vi "Point To Row Column.vi"(8 "error in (no error)":errorcluster, 10 "Point":T2, 11 "DigitalTable in":refnum<class "DigitalTable.lvclass">) -> (0 "error out":errorcluster, 1 "Cell Position":T1, 2 "In Bounds?":bool, 3 "DigitalTable out":refnum<class "DigitalTable.lvclass">)   [LabVIEW 2023, in "DigitalTable.lvclass"]
doc: "Converts a pixel coordinate to a row-column pair in the coordinates of the control. This method also returns whether the point is inside the bounds of the content rectangle.\n\n <b>Note</b> The Point to Row Column method does not return an error for points that lie within a control but outside of the actual cell area for that control, such as the scroll bar. Use the InBounds parameter to verify that a point lies within the cell area of a control.\n\nQControl Class wrapper around the <b>DigitalTable : Point to Row Column Method</b>.\n<b> </b> <b> </b>\n©2016 Q Software Innovations, LLC (QSI)\nwritten by Quentin Alldredge\nproduced in LabVIEW 2015\n\nsupport@qsoftwareinnovations.com\nwww.qsoftwareinnovations.com\n\nAll rights reserved.\n\nRedistribution and use in source and binary forms, with or without modification, are permitted provided that the following conditions are met:\n\n * Redistributions of source code must retain the above copyright notice, this list of conditions and the following disclaimer.\n * Redistributions in binary form must reproduce the above copyright notice, this list of conditions and the following disclaimer in the documentation and/or other materials provided with the distribution.\n * Neither the name of Q Software Innovations, LLC. nor the names of its contributors may be used to endorse or promote products derived from this software without specific prior written permission.\n\nTHIS SOFTWARE IS PROVIDED BY THE COPYRIGHT HOLDERS AND CONTRIBUTORS \"AS IS\" AND ANY EXPRESS OR IMPLIED WARRANTIES, INCLUDING, BUT NOT LIMITED TO, THE IMPLIED WARRANTIES OF MERCHANTABILITY AND FITNESS FOR A PARTICULAR PURPOSE ARE DISCLAIMED. IN NO EVENT SHALL THE COPYRIGHT OWNER OR CONTRIBUTORS BE LIABLE FOR ANY DIRECT, INDIRECT, INCIDENTAL, SPECIAL, EXEMPLARY, OR CONSEQUENTIAL DAMAGES (INCLUDING, BUT NOT LIMITED TO, PROCUREMENT OF SUBSTITUTE GOODS OR SERVICES; LOSS OF USE, DATA, OR PROFITS; OR BUSINESS INTERRUPTION) HOWEVER CAUSED AND ON ANY THEORY OF LIABILITY, WHETHER IN CONTRACT, STRICT LIABILITY, OR TORT (INCLUDING NEGLIGENCE OR OTHERWISE) ARISING IN ANY WAY OUT OF THE USE OF THIS SOFTWARE, EVEN IF ADVISED OF THE POSSIBILITY OF SUCH DAMAGE."
uses:
  DigitalTable.lvclass
  <vilib>/Utility/miscctls.llb/LVPositionTypeDef.ctl
  <vilib>/Utility/miscctls.llb/LVRowAndColumnTypeDef.ctl
  DigitalTable.lvclass/DigitalTable.ctl
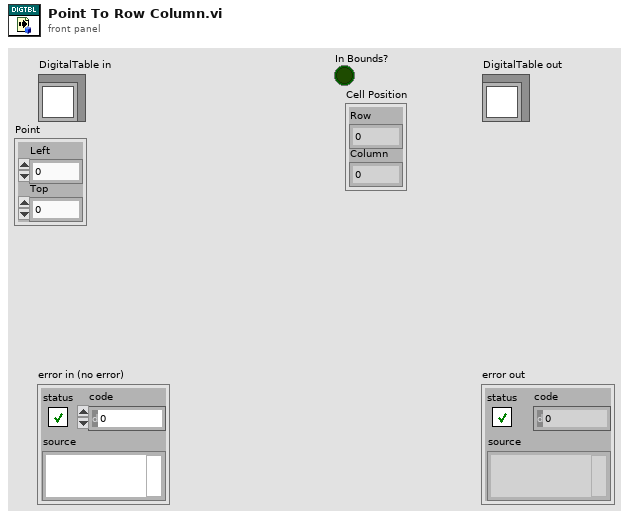
[diagram p1: front panel]
types:
  T1 = typedef "LVRowAndColumnTypeDef.ctl" = cluster{"Row":i32, "Column":i32}
  T2 = typedef "LVPositionTypeDef.ctl" = cluster{"Left":i32, "Top":i32}
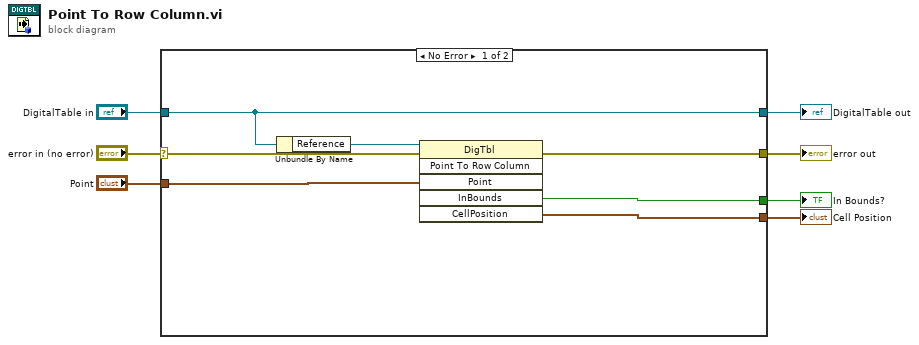
[diagram p0: block diagram]
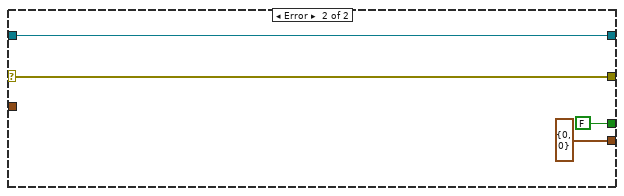
[diagram p2: hidden frame]
diagram:
  n1 = case shown="No Error" "error in (no error)" {
    selector: "error in (no error)" -> [w14 w18]
    tunnel: [w13 w18] -> w6
    tunnel: [w12 w17] -> w4
    tunnel: "DigitalTable in" -> [w12 w17]
    tunnel: "Point" -> [w10 _]
    tunnel: [w9 FALSE ("InBounds")] -> w2
    tunnel: [w8 T1 {"Row"=0, "Column"=0} ("CellPosition")] -> w1
    frame No Error {
      n2 = Unbundle By Name(w12) -> ("Reference"=w11:refnum<vi>)
      n3 = invoke class="DigTbl" method="Point To Row Column"(reference=w11, error in=w14, "Point"=w10) -> (error out=w13:errorcluster, "InBounds"=w9:bool, "CellPosition"=w8:T1)  [unwired: 3 in, 3 out]
    }
    frame Error {
    }
  }
  "error out" <- w6
  "DigitalTable out" <- w4
  "In Bounds?" <- w2
  "Cell Position" <- w1
